vi "Main Loop.vi"(8 "error in (no error)":errorcluster, 10 "Chart Notifier":refnum<notifier>, 11 "Message Queues":T1) -> (0 "error out":errorcluster)   [LabVIEW 2018, in "Feed Module.lvlib" / "Feed Module Engine.lvlib"]
uses:
  Feed Module Engine.lvlib
  Feed Module/Controls/Feed Message Queues.ctl
  support/Message Queue/Message Cluster.ctl
  State Cluster.ctl
  State Enum.ctl
  Feed Module/Controls/Feed Module Settings Cluster.ctl
  Ismatec ISM 831C/Controls/Ismatech Settings Cluster.ctl
  Masterflex 7550-30/Controls/Settings Cluster.ctl
  Mettler Toledo/Controls/Settings Cluster.ctl
  Bronkhorst M13 Flow Meter/Settings Cluster.ctl
  PID 2 Parameters Cluster.ctl
  PID Input Enum.ctl
  PID 2 Output Enum.ctl
  Tacmina QI/Tacmina QI DAQ Setting.ctl
  KNF Pump/Settings Cluster plus SIMDOS.ctl
  ASIA Pump/Pump Settings.ctl
  VICI M50 Party Mode/Settings Cluster.ctl
  FLOM Pump/Settings Cluster.ctl
  SSI PR Class/SSI PR Settings Cluster.ctl
  PID 1 Parameters Cluster.ctl
  Feed Module/Controls/Feed Module Display.ctl
  Config Module/Controls/OP Window Display.ctl
  <vilib>/Platform/TimedLoop/XDataNode/timing_clust.ctl
  <vilib>/Platform/TimedLoop/XDataNode/nitl_modes.ctl
  <vilib>/Platform/TimedLoop/XDataNode/wakeup.ctl
  Tag VIs/Tag FGV Operation Enum.ctl
  support/Message Queue/Enqueue Message (Single).vi
  <vilib>/Utility/error.llb/Error Cluster From Error Code.vi
  <vilib>/Platform/TimedLoop/XDataNode/XDataNode.xnode
  <vilib>/ErrorRing/Error Ring.xnode
  support/Message Queue/Message Queue.lvlib
  <vilib>/Platform/TimedLoop/XDataNode/XDNodeRunTimeDep.lvlib
  Feed Module/Feed Module.lvlib
  Ismatec ISM 831C/Ismatec ISM 831C.lvlib
  Masterflex 7550-30/Masterflex 7550-30.lvlib
  Bronkhorst M13 Flow Meter/Bronkhorst M13 Flow Meter.lvlib
  Mettler Toledo/Mettler Toledo.lvlib
  Tacmina QI/Tacmina QI.lvlib
  Shared Variables/Dynamic Shared Variables.lvlib
  KNF Pump/KNF SIMDOS.lvlib
  ASIA Pump.lvlib
  VICI M50 Party Mode/VICI M6 M50 Party Mode.lvlib
  FLOM Pump/FLOM Pump.lvlib
  SSI PR Class/SSI PR Pump.lvlib
  support/Support Library.lvlib
panel:
  out "Period (s)":dbl format="%_4g"
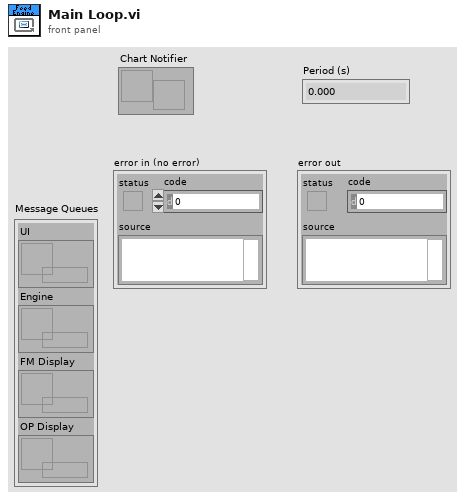
[diagram p1: front panel]
types:
  T1 = typedef "Feed Module.lvlib/Feed Message Queues.ctl" = cluster{"UI":refnum<queue>, "Engine":refnum<queue>, "FM Display":refnum<queue>, "OP Display":refnum<queue>}
  T2 = typedef "XDNodeRunTimeDep.lvlib/timing_clust.ctl" = cluster{"Expected End [f-1]":u64, "Actual End [f-1]":u64, "Finished Late? [f-1]":bool, "Expected End [i-1]":u64, "Actual End [i-1]":u64, "Finished Late? [i-1]":bool, "Expected Start [i]":u64, "Actual Start [i]":u64, "Expected Start [f]":u64, "Actual Start [f]":u64, "Source Name":string, "Structure Name":string, "Period":i64, "Deadline":i64, "Offset":i64, "Start":i64, "Priority":i32, "Timeout":i32, "Mode":T3, "Wakeup Reason":T4, "Error":errorcluster, "Source Type":string, "Secondary Source Type":string, "Global End Time":u64, "Global Start Time":u64, "Frame Duration":u64, "Iteration Duration":u64, "Assigned CPU":i32, "I/O Scan Engine Mode":u32}
  T3 = typedef "XDNodeRunTimeDep.lvlib/nitl_modes.ctl" = enum32{"No Change", "Process missed periods, maintain original phase", "Discard missed periods, maintain original phase", "Process missed periods, ignore original phase", "Discard missed periods, ignore original phase"}
  T4 = typedef "XDNodeRunTimeDep.lvlib/wakeup.ctl" = enum32{"Normal", "Aborted", "Asynchronous wakeup", "Timing source error", "Timed loop error", "Timeout"}
  T5 = cluster{"enable? (F)":bool, "name":string, "alarm on":bool, "priority":u32, "ack type":enum16{"Auto", "User", "None", "Each Occurrence"}, "area":string, "description":string, "log? (T)":bool}
  T6 = typedef "Tag FGV Operation Enum.ctl" = enum16{"Init", "Set Notification Queue", "Create Tag", "Commit", "Write Tag (Numeric)", "Write Tag (Boolean)", "Read All Tags", "Read One Tag", "Delete Tag Category", "Set Alarm Parameters (Numeric)", "Set Alarm Parameters (Boolean)", "Enable All Alarms", "Disable All Alarms", "Delete All Tags", "Read Alarms", "Ack Alarm"}
  T7 = enum32{"u32BitField", "bool", "double", "string", "int8", "uint8", "int16", "uint16", "int32", "uint32", "int64", "uint64", "single", "double waveform", "int16 waveform", "array of boolean", "array of int8", "array of uint8", "array of int16", "array of uint16", "array of int32", "array of uint32", "array of int64", "array of uint64", "array of single", "array of double", "array of double waveform", "array of int16 waveform", "array of string", "variant", "timestamp", "fixed point", "custom"}
  T8 = typedef "Feed Module.lvlib/Feed Module Engine.lvlib/State Enum.ctl" = enum16{"Measuring", "Idle", "Paused"}
  T9 = typedef "Feed Module.lvlib/OP Window Display.ctl" = cluster{"Flow":dbl, "Manual":dbl, "Pump Status":u16}
  T10 = typedef "Feed Module.lvlib/Feed Module Display.ctl" = cluster{"Flow":dbl, "Density":dbl, "FL Temp":dbl, "Scale Value":dbl, "Pump On?":enum16{"Off", "On", "Not Initialized"}, "Cycle Period":dbl, "Input Device":T11, "Output":T12, "Pump's Pressure":dbl, "Pump's Flow ":dbl}
  T11 = typedef "PID Input Enum.ctl" = enum16{"Default", "Bronkhorst M13", "Bronkhorst M14", "Scale Rate of Change"}
  T12 = typedef "PID 2 Output Enum.ctl" = enum16{"Default", "Ismatec ISM 831C", "Masterflex 7550-30", "VICI", "Tacmina QI", "KNF SIMDOS", "ASIA Type C", "FLOM UI-22-11", "SSI PR"}
  T13 = typedef "Feed Module.lvlib/Feed Module Engine.lvlib/State Cluster.ctl" = cluster{"State":T8, "Start Time":timestamp, "Configuration":T14, "Current Time":timestamp, "PID 1 Parameters":T26, "First Iteration":bool, "Data":cluster{"Flowmeter Output":dbl, "Density":dbl, "FL Temp":dbl, "Scale Output (g)":dbl, "Scale Rate of Change (g/min)":dbl, "PID 1 Output":dbl, "PID 2 Process Variable":dbl, "PID 2 output":dbl, "Pump Flow":dbl, "Pump Pressure":dbl}, "Process Name":string, "Pump On?":enum16{"Off", "On", "Not Initialized"}, "Input Error":bool, "Output Error":bool, "Log Started":bool, "Current Setpoint":dbl}
  T14 = typedef "Feed Module.lvlib/Feed Module Settings Cluster.ctl" = cluster{"Cycle Period":dbl, "Ismatech":T15, "Masterflex":T16, "Mettler":T17, "Bronkhorst M13 Flow Meter":T18, "PID 2 Parameters":T19, "Manual Entry":dbl, "Auto?":bool, "output range":cluster{"output high":dbl, "output low":dbl}, "Bronkhorst M14":T17, "Tacmina Settings":T20, "KNF SIMDOS Settings":T21, "ASIA Pump C":T22, "VICI Settings":T23, "FLOM Settings":T24, "SSI PR Settings":T25}
  T15 = typedef "Ismatec ISM 831C.lvlib/Ismatech Settings Cluster.ctl" = cluster{"VISA resource name":refnum<visa-resource-name>, "Simulated?":bool, "Pump Number":dbl, "Reverse?":bool}
  T16 = typedef "Masterflex 7550-30.lvlib/Settings Cluster.ctl" = cluster{"VISA resource name":refnum<visa-resource-name>, "Simulated?":bool, "Pump Number":dbl, "Reverse?":bool}
  T17 = typedef "Mettler Toledo.lvlib/Settings Cluster.ctl" = cluster{"VISA resource name":refnum<visa-resource-name>, "Simulated?":bool}
  T18 = typedef "Bronkhorst M13 Flow Meter.lvlib/Settings Cluster.ctl" = cluster{"VISA resource name":refnum<visa-resource-name>, "Simulated?":bool}
  T19 = typedef "PID 2 Parameters Cluster.ctl" = cluster{"Input Device":T11, "Output Device":T12, "Setpoint":dbl, "PID gains":cluster{"proportional gain (Kc)":dbl, "integral time (Ti, min)":dbl, "derivative time (Td, min)":dbl}}
  T20 = typedef "Tacmina QI.lvlib/Tacmina QI DAQ Setting.ctl" = cluster{"Analog DAQ Task":refnum<k21>, "Digital DAQ Task":refnum<k21>}
  T21 = typedef "KNF SIMDOS.lvlib/Settings Cluster plus SIMDOS.ctl" = cluster{"VISA resource name":refnum<visa-resource-name>, "Simulated?":bool}
  T22 = typedef "ASIA Pump.lvlib/Pump Settings.ctl" = cluster{"ASIA Pump #":i32, "channel":i32, "Simulated":bool}
  T23 = typedef "VICI M6 M50 Party Mode.lvlib/Settings Cluster.ctl" = cluster{"VISA resource name":refnum<visa-resource-name>, "Simulated?":bool, "Pump Letter":string, "Reverse?":bool}
  T24 = typedef "FLOM Pump.lvlib/Settings Cluster.ctl" = cluster{"VISA resource name":refnum<visa-resource-name>, "Simulated?":bool, "Pump Number":dbl}
  T25 = typedef "SSI PR Pump.lvlib/SSI PR Settings Cluster.ctl" = cluster{"VISA resource name":refnum<visa-resource-name>, "Simulated?":bool}
  T26 = typedef "PID 1 Parameters Cluster.ctl" = cluster{"Setpoint":dbl, "PID gains":cluster{"proportional gain (Kc)":dbl, "integral time (Ti, min)":dbl, "derivative time (Td, min)":dbl}}
  T27 = cluster{"Flowmeter Output":dbl, "Density":dbl, "FL Temp":dbl, "Scale Output (g)":dbl, "Scale Rate of Change (g/min)":dbl, "PID 1 Output":dbl, "PID 2 Process Variable":dbl, "PID 2 output":dbl, "Pump Flow":dbl, "Pump Pressure":dbl}
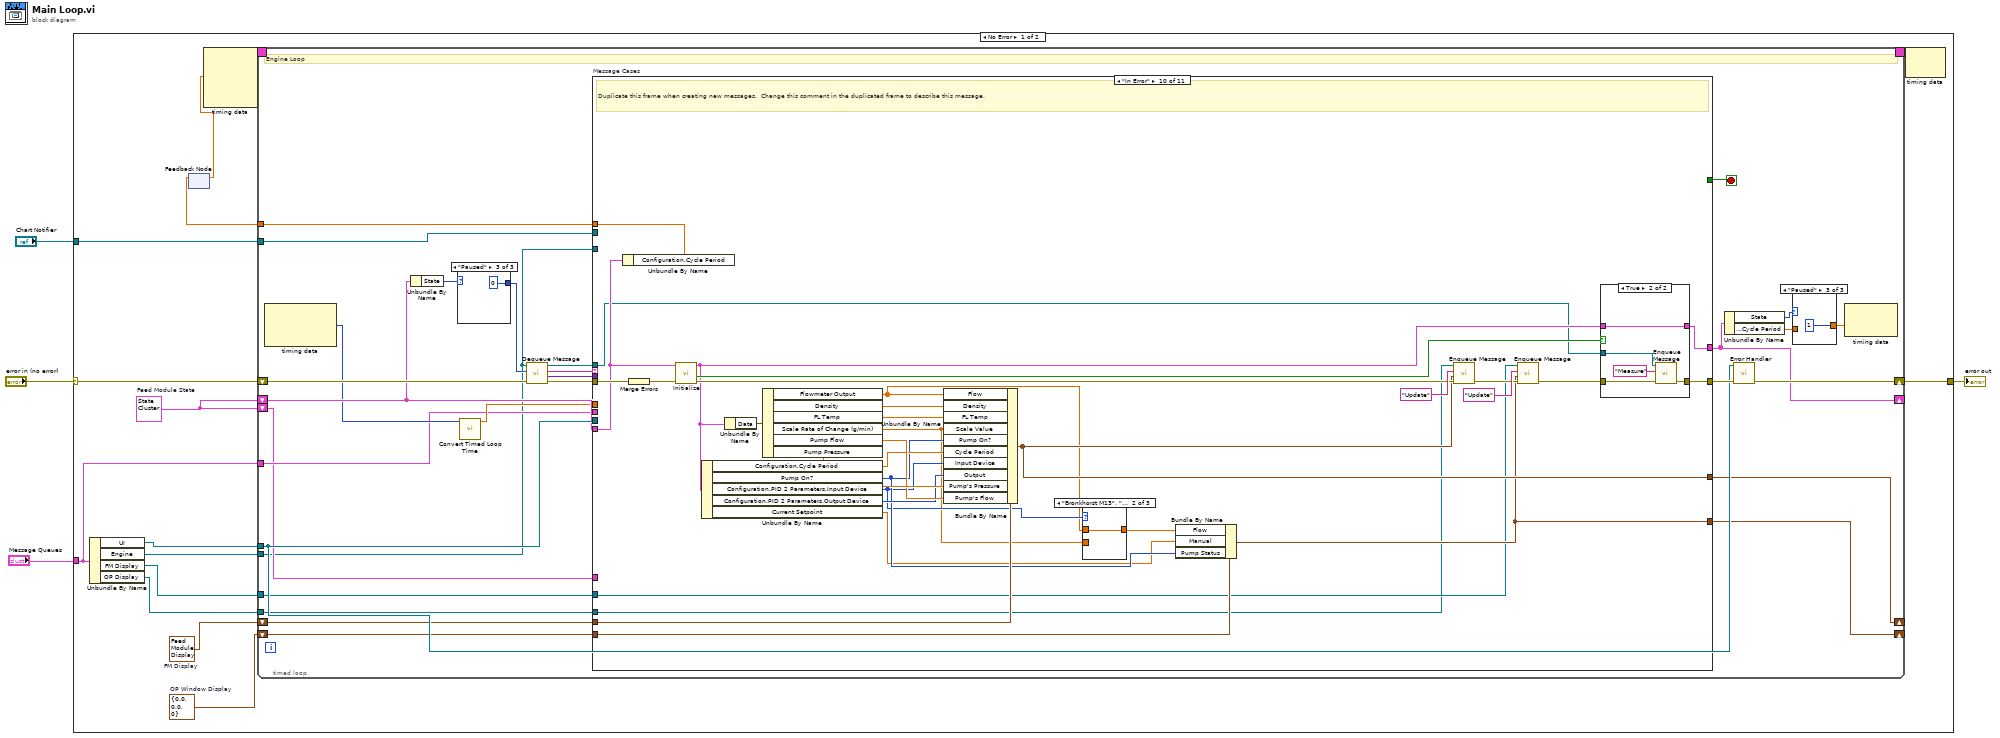
[diagram p0: block diagram]
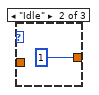
[diagram p3: hidden frame]
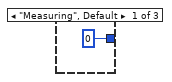
[diagram p4: hidden frame]
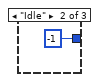
[diagram p5: hidden frame]
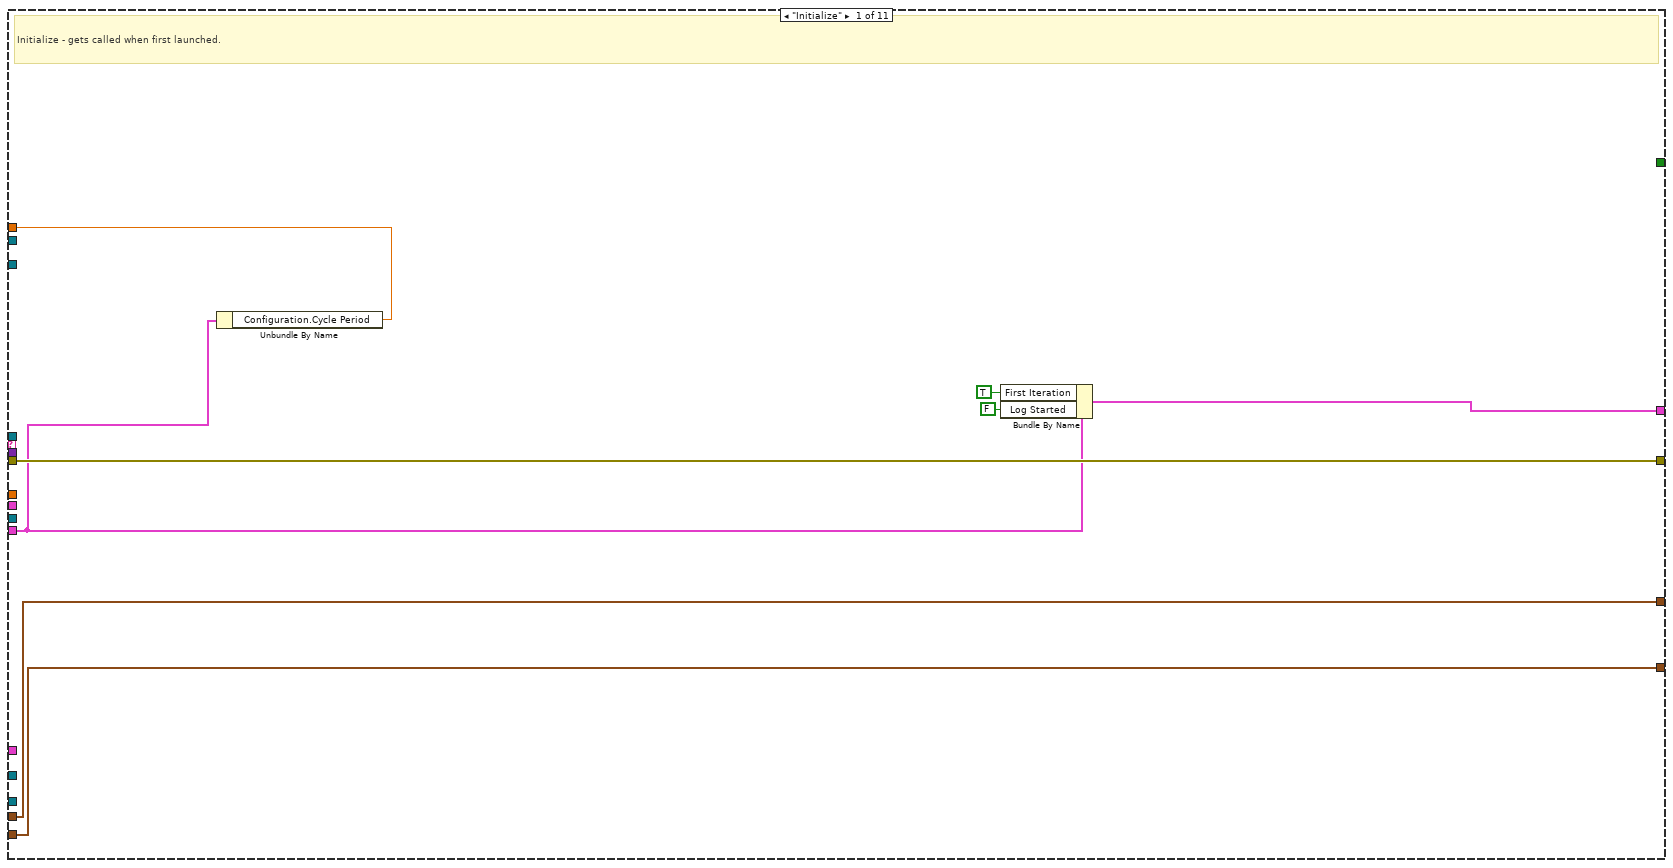
[diagram p6: hidden frame]
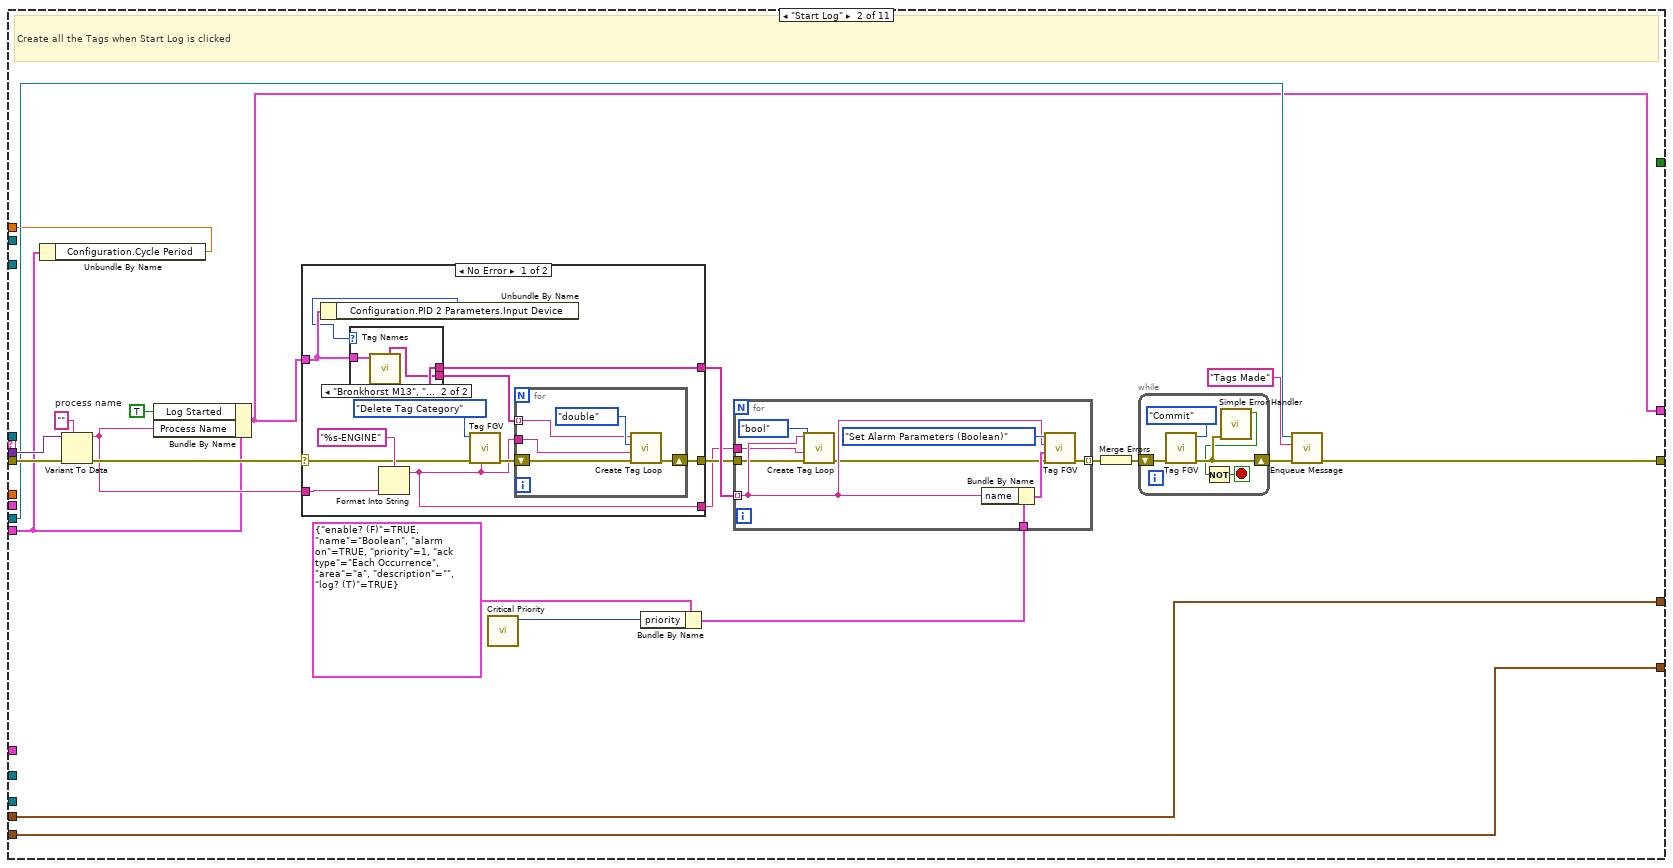
[diagram p7: hidden frame]
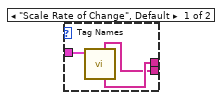
[diagram p8: hidden frame]
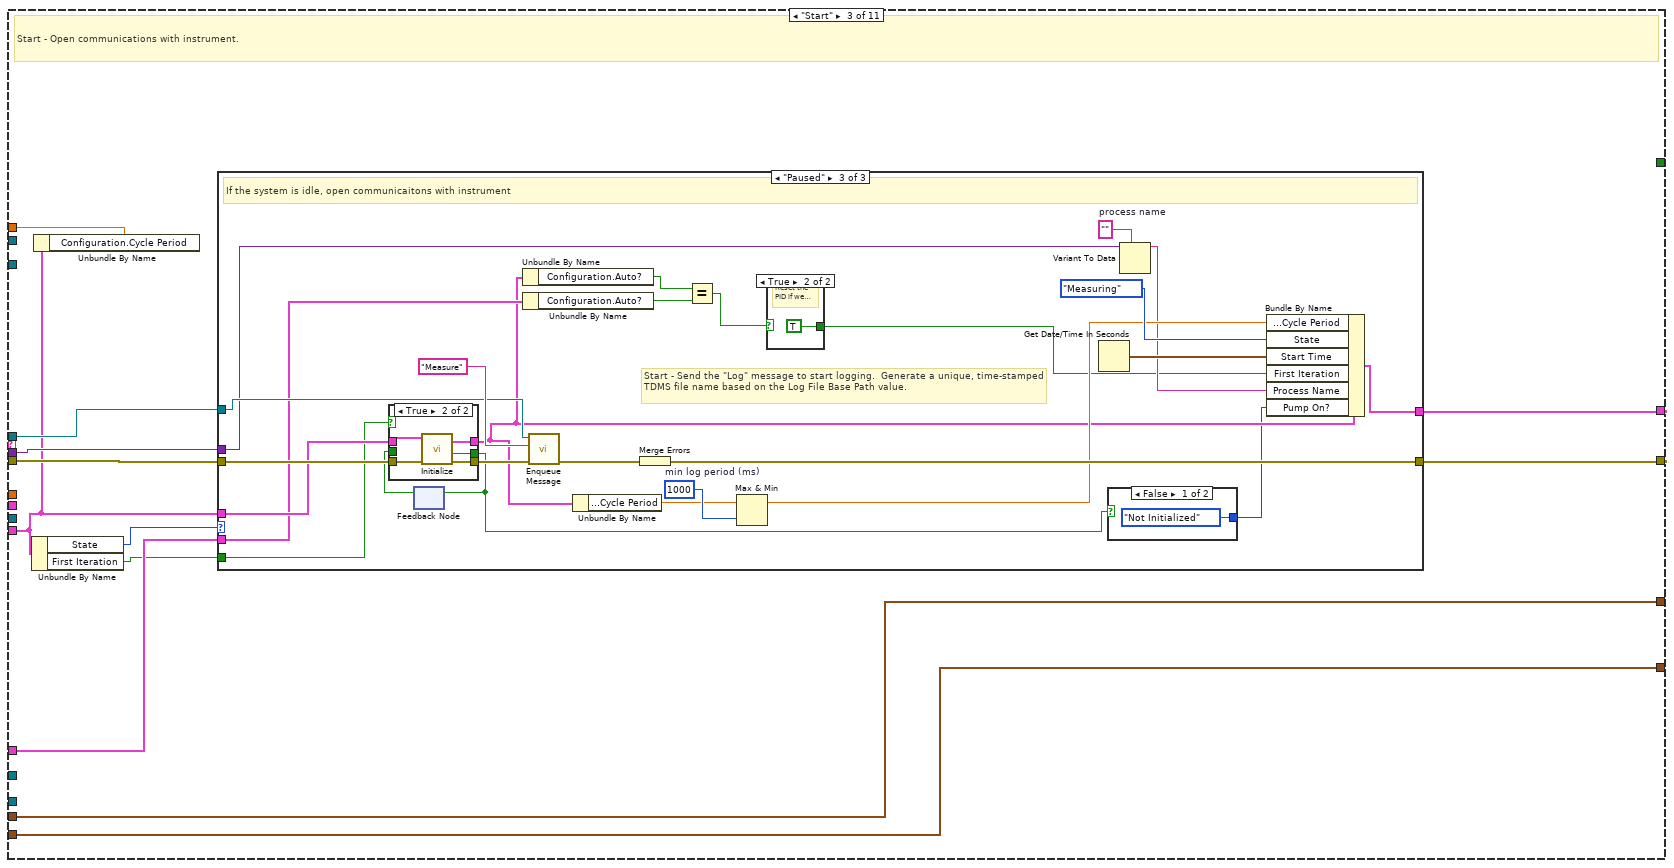
[diagram p10: hidden frame]
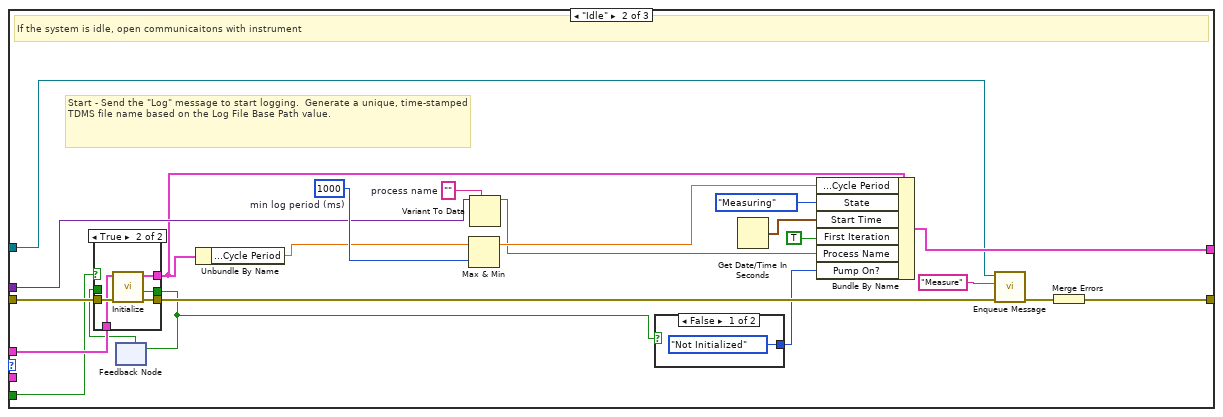
[diagram p12: hidden frame]
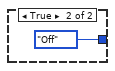
[diagram p14: hidden frame]
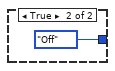
[diagram p16: hidden frame]
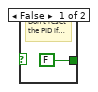
[diagram p17: hidden frame]
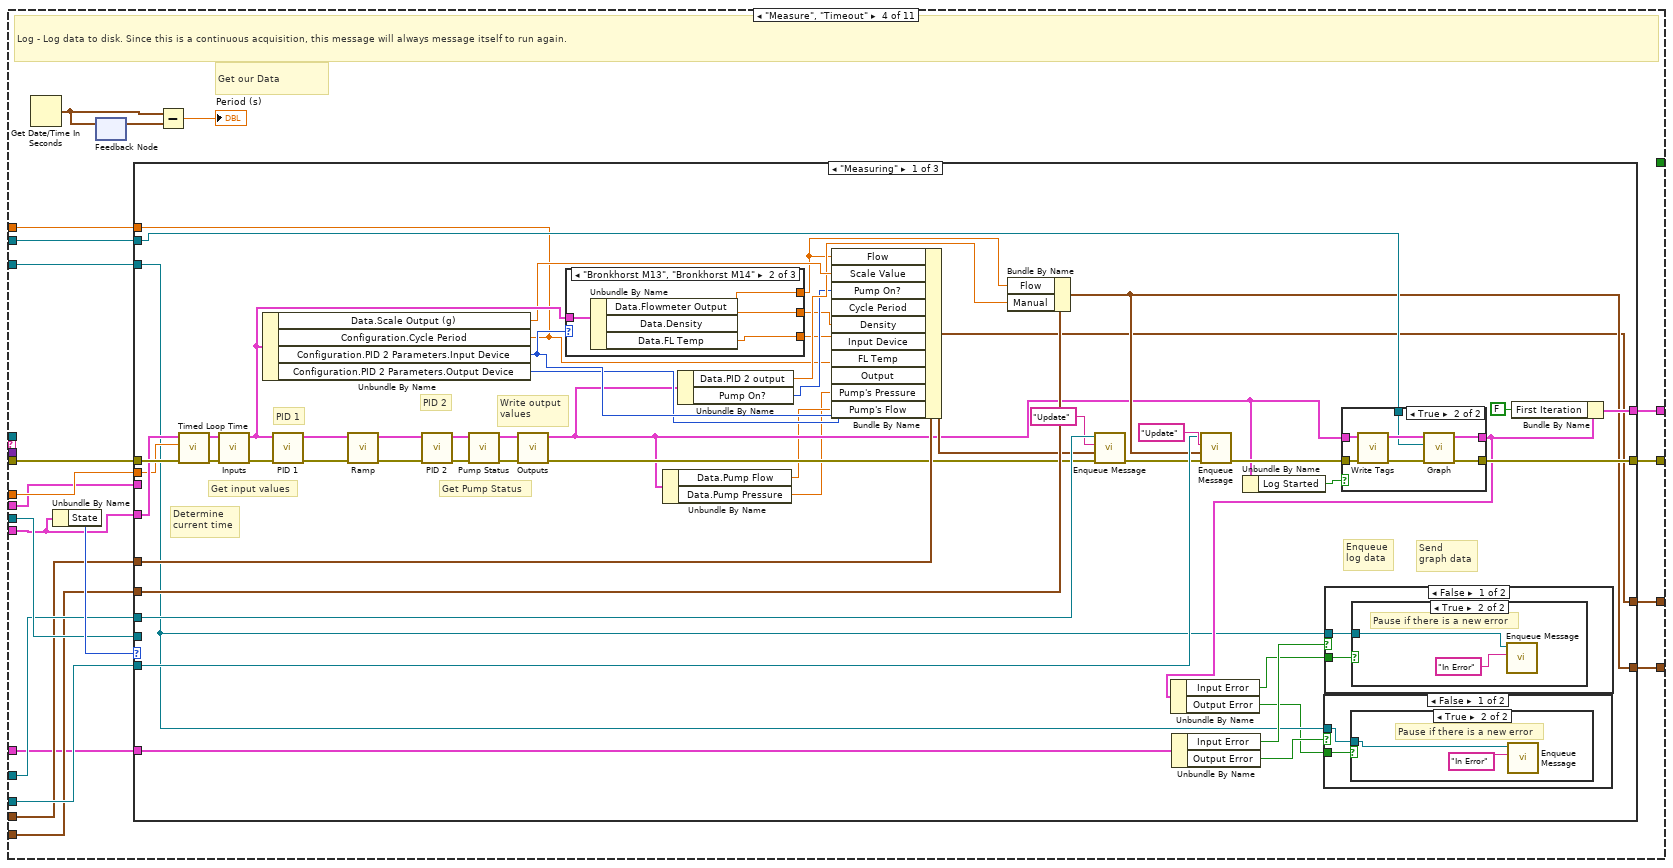
[diagram p18: hidden frame]
diagram:
  n1 = case shown="No Error" "error in (no error)" {
    selector: "error in (no error)" -> [w18 w566]
    tunnel: "Message Queues" -> [w14 _]
    tunnel: [w19 w566] -> w3
    tunnel: "Chart Notifier" -> [w12 _]
    frame No Error {
      w9 = T9 {"Flow"=0.0, "Manual"=0.0, "Pump Status"=0}  # OP Window Display
      w7 = T10 {"Flow"=0.0, "Density"=0.0, "FL Temp"=0.0, "Scale Value"=0.0, "Pump On?"=enum."Off", "Cycle Period"=500.0, "Input Device"=enum."Bronkhorst M13", "Output"=enum."Default", "Pump's Pressure"=0.0, "Pump's Flow "=0.0}  # FM Display
      w10 = T13 {"State"=enum."Idle", "Start Time"=timestamp(0 s since 1904-01-01), "Configuration"={"Cycle Period"=0.0, "Ismatech"={"VISA resource name"="", "Simulated?"=FALSE, "Pump Number"=1.0, "Reverse?"=FALSE}, "Masterflex"={"VISA resource name"="", "Simulated?"=FALSE, "Pump Number"=1.0, "Reverse?"=FALSE}, "Mettler"={"VISA resource name"="", "Simulated?"=FALSE}, "Bronkhorst M13 Flow Meter"={"VISA resource name"="", "Simulated?"=FALSE}, "PID 2 Parameters"={"Input Device"=enum."Bronkhorst M13", "Output Device"=enum."Ismatec ISM 831C", "Setpoint"=0.0, "PID gains"={"proportional gain (Kc)"=1.0, "integral time (Ti, min)"=0.01, "derivative time (Td, min)"=0.0}}, "Manual Entry"=0.0, "Auto?"=TRUE, "output range"={"output high"=100.0, "output low"=0.0}, "Bronkhorst M14"={"VISA resource name"="", "Simulated?"=FALSE}, "Tacmina Settings"={"Analog DAQ Task"="", "Digital DAQ Task"=""}, "KNF SIMDOS Settings"={"VISA resource name"="", "Simulated?"=TRUE}, "ASIA Pump C"={"ASIA Pump #"=0, "channel"=0, "Simulated"=FALSE}, "VICI Settings"={"VISA resource name"="", "Simulated?"=FALSE, "Pump Letter"="", "Reverse?"=FALSE}, "FLOM Settings"={"VISA resource name"="", "Simulated?"=TRUE, "Pump Number"=0.0}, "SSI PR Settings"={"VISA resource name"="", "Simulated?"=FALSE}}, "Current Time"=timestamp(0 s since 1904-01-01), "PID 1 Parameters"={"Setpoint"=0.0, "PID gains"={"proportional gain (Kc)"=1.0, "integral time (Ti, min)"=0.01, "derivative time (Td, min)"=0.0}}, "First Iteration"=FALSE, "Data"={"Flowmeter Output"=0.0, "Density"=0.0, "FL Temp"=0.0, "Scale Output (g)"=0.0, "Scale Rate of Change (g/min)"=0.0, "PID 1 Output"=0.0, "PID 2 Process Variable"=0.0, "PID 2 output"=0.0, "Pump Flow"=0.0, "Pump Pressure"=0.0}, "Process Name"="", "Pump On?"=enum."Off", "Input Error"=FALSE, "Output Error"=FALSE, "Log Started"=FALSE, "Current Setpoint"=0.0}  # Feed Module State
      n2 = Unbundle By Name(w14) -> ("UI"=w17:refnum<queue>, "Engine"=w13:refnum<queue>, "FM Display"=w11:refnum<queue>, "OP Display"=w8:refnum<queue>)
      n3 = feedback #1() -> (w5:dbl)  [unwired: 1 in]
      n4 = node-c288(w5) -> (w16:T2)  [unwired: 3 in]
      n5 = timed-loop {
        tunnel: w13 -> [w23]
        shift-right: [w37] -> _
        shift-left: w10 -> [w40]
        shift-right: [w42] -> w19
        shift-left: w18 -> [w48]
        tunnel: w17 -> [w41]
        timing: w16 -> [_]
        timing-out: [_] -> w15
        tunnel: w14 -> [w31]
        tunnel: w12 -> [w30]
        tunnel: w11 -> [w29]
        tunnel: w8 -> [w28]
        shift-right: [w27] -> _
        shift-left: w7 -> [w21]
        shift-right: [w26] -> _
        shift-left: w9 -> [w22]
        shift-left: w10 -> [w25]
        tunnel: [w20] -> w6
        stop <- w24 stop-if-true
        # "Engine Loop"
        n6 = node-c288() -> (w33:i64)  [unwired: 1 in, 2 out]
        n7 = Unbundle By Name(w40) -> ("State"=w39:T8)
        n8 = case shown="\"Paused\"" w39 {
          tunnel: [0 ("timeout in ms (-1)") -1 ("timeout in ms (-1)") 0 ("timeout in ms (-1)")] -> w38
          frame "Measuring", Default {
          }
          frame "Idle" {
          }
          frame "Paused" {
          }
        }
        n9 = call "Convert Timed Loop Time.vi"("Actual Start [i]"=w33) -> ("ET since start (s)"=w32:dbl)  [unwired: 10 in]
        n10 = call "Dequeue Message.vi"("error in (no error)"=w48, "timeout in ms (-1)"=w38, "Message Queue"=w23) -> ("error out"=w47:errorcluster, "Message Data"=w45:variant, "Message"=w46:string, "dup Message Queue"=w44:refnum<queue>)  [unwired: 5 in]
        n11 = case "Message Cases" shown="\"In Error\"" w46 {
          selector: w46 -> [_ _ _ _ _ _ _ _ _ _ w553]
          tunnel: w44 -> [_ _ w138 _ w413 _ _ w489 _ w502 _]
          tunnel: w47 -> [w67 w86 w137 w229 w400 w429 w481 w492 w501 w534 _]
          tunnel: [w67 w73 w139 w230 w405 w433 w475 w494 w500 w530 w554] -> w43
          tunnel: w40 -> [w61 w70 w129 w227 w399 w426 w477 w484 w497 w529 w550]
          tunnel: [w64 w72 w136 w228 w401 w431 w474 w484 w497 w531 w550] -> w37
          tunnel: [_ _ _ _ _ _ _ TRUE _ _ _] -> w24
          tunnel: w45 -> [_ w87 w134 _ _ _ w482 _ _ _ _]
          tunnel: w41 -> [_ w74 _ w231 w412 w442 _ w493 _ _ _]
          tunnel: w32 -> [_ _ _ w226 _ _ _ _ _ _ _]
          tunnel: w31 -> [_ _ _ w225 _ _ _ _ _ _ _]
          tunnel: w30 -> [_ _ _ w221 _ _ _ _ _ _ _]
          tunnel: w29 -> [_ _ _ w220 w403 w436 _ _ _ w504 _]
          tunnel: w28 -> [_ _ _ w219 w404 w435 _ _ _ w503 _]
          tunnel: w21 -> [w65 w90 w133 w218 w410 w440 w479 w486 w499 w522 w552]
          tunnel: [w65 w90 w133 w217 w410 w440 w479 w486 w499 w512 w552] -> w27
          tunnel: w22 -> [w66 w89 w132 w216 w402 w432 w478 w485 w498 w521 w551]
          tunnel: [w66 w89 w132 w215 w402 w432 w478 w485 w498 w505 w551] -> w26
          tunnel: w25 -> [_ _ w131 w214 _ _ _ _ _ _ _]
          tunnel: w23 -> [_ _ _ w213 _ _ _ _ _ _ _]
          tunnel: [w62 w71 w128 w212 w398 w425 w473 w483 w496 w528 w549] -> w20
          frame "Initialize" {
            # "Initialize - gets called when first launched."
            n12 = Unbundle By Name(w61) -> ("Configuration.Cycle Period"=w62:dbl)
            n13 = Bundle By Name(cluster=w61, "First Iteration"=TRUE, "Log Started"=FALSE) -> (w64:T13)
          }
          frame "Start Log" {
            w88 = ""  # process name
            # "Create all the Tags when Start Log is clicked"
            n14 = Unbundle By Name(w70) -> ("Configuration.Cycle Period"=w71:dbl)
            n15 = Variant To Data(error in=w86, type=w88, Variant=w87) -> (data=w84:string, error out=w85:errorcluster)
            n16 = Bundle By Name(cluster=w70, "Log Started"=TRUE, "Process Name"=w84) -> (w72:T13)
            n17 = case shown="No Error" w85 {
              selector: w85 -> [w112 w127]
              tunnel: [w115 w127] -> w79
              tunnel: w84 -> [w110 _]
              tunnel: [w109 _] -> w80
              tunnel: [w108 _] -> w77
              tunnel: w72 -> [w106 _]
              frame No Error {
                n18 = Unbundle By Name(w106) -> ("Configuration.PID 2 Parameters.Input Device"=w105:T11)
                n19 = case shown="\"Bronkhorst M13\", \"Bronkhorst M14\"" w105 {
                  tunnel: [w117 w121] -> w109
                  tunnel: [w116 w119] -> w107
                  tunnel: w106 -> [w118 w120]
                  frame "Scale Rate of Change", Default {
                    n20 = call "Tag Names.vi"("State in"=w118) -> ("All Boolean Tags"=w117:string[], "All  Numeric Tags"=w116:string[])  [unwired: 6 in, 3 out]
                  }
                  frame "Bronkhorst M13", "Bronkhorst M14" {
                    n21 = call "Tag Names.vi"("State in"=w120) -> ("All Boolean Tags"=w121:string[], "All  Numeric Tags"=w119:string[])  [unwired: 6 in, 3 out]
                  }
                }
                n22 = Format Into String(format string="%s-ENGINE", w110) -> (resulting string=w108:string)  [unwired: 2 in, 1 out]
                n23 = call "Tag FGV.vi"("Tag Category"=w108, "error in (no error)"=w112, "Operation"=Tag_FGV_Operation_Enum."Delete Tag Category") -> ("error out"=w111:errorcluster)  [unwired: 3 in, 5 out]
                n24 = for {
                  tunnel: w107 -> [w123] mode=indexing
                  shift-right: [w122] -> w115
                  shift-left: w111 -> [w125]
                  tunnel: w108 -> [w124]
                  n25 = call "Create Tag Loop.vi"("error in (no error)"=w125, "Tag Category"=w124, "data type"=T7."double", "Tag Name"=w123) -> ("error out"=w122:errorcluster)  [unwired: 7 in]
                }
              }
              frame Error {
              }
            }
            n26 = call "Critical Priority.vi"() -> ("critical priority"=w82:i32)  [unwired: 11 in]
            n27 = Bundle By Name(cluster=T5 {"enable? (F)"=TRUE, "name"="Boolean", "alarm on"=TRUE, "priority"=1, "ack type"=enum."Each Occurrence", "area"="a", "description"="", "log? (T)"=TRUE} ("Boolean alarm settings"), "priority"=w82) -> (w81:T5)
            n28 = for {
              tunnel: w81 -> [w104]
              tunnel: [w103] -> w78 mode=indexing
              tunnel: w80 -> [w99] mode=indexing
              tunnel: w79 -> [w97]
              tunnel: w77 -> [w98]
              n29 = call "Create Tag Loop.vi"("error in (no error)"=w97, "Tag Category"=w98, "data type"=T7."bool", "Tag Name"=w99) -> ("error out"=w96:errorcluster)  [unwired: 7 in]
              n30 = Bundle By Name(cluster=w104, "name"=w99) -> (w102:T5)
              n31 = call "Tag FGV.vi"("error in (no error)"=w96, "Data"=w102, "Tag Name"=w99, "Operation"=Tag_FGV_Operation_Enum."Set Alarm Parameters (Boolean)") -> ("error out"=w103:errorcluster)  [unwired: 2 in, 5 out]
            }
            n32 = Merge Errors(w78) -> (w69:errorcluster)
            n33 = while {
              shift-right: [w93] -> w68
              shift-left: w69 -> [w94]
              stop <- w91 stop-if-true
              n34 = call "Tag FGV.vi"("error in (no error)"=w94, "Operation"=Tag_FGV_Operation_Enum."Commit") -> ("error out"=w93:errorcluster)  [unwired: 4 in, 5 out]
              n35 = call <vilib>:"Simple Error Handler.vi"("error in (no error)"=w93) -> ("error?"=w92:bool)  [unwired: 4 in, 4 out]
              n36 = Not(x=w92) -> (.not. x?=w91:bool)
            }
            n37 = call-poly "Enqueue Message.vi"("error in (no error)"=w68, "Message"="Tags Made", "Message Queue"=w74) -> ("error out"=w73:errorcluster)  [unwired: 7 in, 1 out]
          }
          frame "Start" {
            # "Start - Open communications with instrument."
            n38 = Unbundle By Name(w129) -> ("State"=w135:T8, "First Iteration"=w130:bool)
            n39 = Unbundle By Name(w129) -> ("Configuration.Cycle Period"=w128:dbl)
            n40 = case shown="\"Paused\"" w135 {
              tunnel: [w140 w163 w199] -> w139
              tunnel: w138 -> [_ w154 w190]
              tunnel: w137 -> [w140 w152 w188]
              tunnel: w129 -> [w141 w151 w187]
              tunnel: [w141 w161 w197] -> w136
              tunnel: w134 -> [_ w149 w185]
              tunnel: w131 -> [_ _ w181]
              tunnel: w130 -> [_ w142 w176]
              frame "Measuring", Default {
                # "The system is already running. Ignore the \"Start\" message."
              }
              frame "Idle" {
                w150 = ""  # process name
                w158 = 1000  # min log period (ms)
                # "Start - Send the \"Log\" message to start logging.  Generate a unique, time-stamped TDMS file name based on the Log File Base Path value."
                # "If the system is idle, open communicaitons with instrument"
                n41 = feedback #2() -> (w144:bool)  [unwired: 1 in]
                n42 = case shown="True" w142 {
                  tunnel: w152 -> [w165 w171]
                  tunnel: w151 -> [w166 w170]
                  tunnel: [w166 w169] -> w147
                  tunnel: [w165 w168] -> w146
                  tunnel: [w164 w167] -> w143
                  tunnel: w144 -> [w164 _]
                  frame False {
                  }
                  frame True {
                    n43 = call "Initialize.vi"("error in (no error)"=w171, "State in"=w170) -> ("error out"=w168:errorcluster, "Pump Initialized"=w167:bool, "State out"=w169:T13)  [unwired: 7 in]
                  }
                }
                n44 = feedback-in #2(w143) -> ()
                n45 = Unbundle By Name(w147) -> ("Configuration.Cycle Period"=w157:dbl)
                n46 = Max & Min(x=w157, y=w158) -> (max(x,y)=w156:dbl)  [unwired: 1 out]
                n47 = Variant To Data(type=w150, Variant=w149) -> (data=w148:string)  [unwired: 1 in, 1 out]
                n48 = case shown="False" w143 {
                  tunnel: [enum16{"Off", "On", "Not Initialized"}."Not Initialized" ("Pump On?") enum16{"Off", "On", "Not Initialized"}."Off" ("Pump On?")] -> w145
                  frame False {
                  }
                  frame True {
                  }
                }
                n49 = Get Date/Time In Seconds() -> (seconds since 1Jan1904=w155:timestamp)
                n50 = Bundle By Name(cluster=w147, "Configuration.Cycle Period"=w156, "State"=State_Enum."Measuring", "Start Time"=w155, "First Iteration"=TRUE, "Process Name"=w148, "Pump On?"=w145) -> (w161:T13)
                n51 = call-poly "Enqueue Message.vi"("error in (no error)"=w146, "Message"="Measure", "Message Queue"=w154) -> ("error out"=w159:errorcluster)  [unwired: 7 in, 1 out]
                n52 = Merge Errors(w159) -> (w163:errorcluster)
              }
              frame "Paused" {
                w186 = ""  # process name
                w194 = 1000  # min log period (ms)
                # "Start - Send the \"Log\" message to start logging.  Generate a unique, time-stamped TDMS file name based on the Log File Base Path value."
                # "If the system is idle, open communicaitons with instrument"
                n53 = feedback #3() -> (w175:bool)  [unwired: 1 in]
                n54 = case shown="True" w176 {
                  tunnel: [w202 w207] -> w189
                  tunnel: w188 -> [w202 w206]
                  tunnel: w187 -> [w201 w205]
                  tunnel: [w201 w204] -> w178
                  tunnel: [w200 w203] -> w174
                  tunnel: w175 -> [w200 _]
                  frame False {
                  }
                  frame True {
                    n55 = call "Initialize.vi"("error in (no error)"=w206, "State in"=w205) -> ("error out"=w207:errorcluster, "Pump Initialized"=w203:bool, "State out"=w204:T13)  [unwired: 7 in]
                  }
                }
                n56 = feedback-in #3(w174) -> ()
                n57 = Unbundle By Name(w178) -> ("Configuration.Auto?"=w182:bool)
                n58 = Unbundle By Name(w181) -> ("Configuration.Auto?"=w180:bool)
                n59 = call-poly "Enqueue Message.vi"("error in (no error)"=w189, "Message"="Measure", "Message Queue"=w190) -> ("error out"=w195:errorcluster)  [unwired: 7 in, 1 out]
                n60 = Unbundle By Name(w178) -> ("Configuration.Cycle Period"=w193:dbl)
                n61 = Merge Errors(w195) -> (w199:errorcluster)
                n62 = Equal?(x=w182, y=w180) -> (x = y?=w183:bool)
                n63 = Max & Min(x=w193, y=w194) -> (max(x,y)=w192:dbl)  [unwired: 1 out]
                n64 = case shown="True" w183 {
                  tunnel: [FALSE ("First Iteration") TRUE ("First Iteration")] -> w179
                  frame False {
                    # "Don't reset the PID if we are switching Auto?"
                  }
                  frame True {
                    # "Reset the PID if we start from paused"
                  }
                }
                n65 = Get Date/Time In Seconds() -> (seconds since 1Jan1904=w191:timestamp)
                n66 = case shown="False" w174 {
                  tunnel: [enum16{"Off", "On", "Not Initialized"}."Not Initialized" ("Pump On?") enum16{"Off", "On", "Not Initialized"}."Off" ("Pump On?")] -> w177
                  frame False {
                  }
                  frame True {
                  }
                }
                n67 = Variant To Data(type=w186, Variant=w185) -> (data=w184:string)  [unwired: 1 in, 1 out]
                n68 = Bundle By Name(cluster=w178, "Configuration.Cycle Period"=w192, "State"=State_Enum."Measuring", "Start Time"=w191, "First Iteration"=w179, "Process Name"=w184, "Pump On?"=w177) -> (w197:T13)
              }
            }
          }
          frame "Measure", "Timeout" {
            # "Get our Data"
            # "Log - Log data to disk. Since this is a continuous acquisition, this message will always message itself to run again."
            n69 = Get Date/Time In Seconds() -> (seconds since 1Jan1904=w223:timestamp)
            n70 = Unbundle By Name(w227) -> ("State"=w232:T8)
            n71 = feedback-in #4(w223) -> ()
            n72 = feedback #4() -> (w224:timestamp)  [unwired: 1 in]
            n73 = case shown="\"Measuring\"" w232 {
              tunnel: w229 -> [w280 w315 w338]
              tunnel: w227 -> [w278 w313 w339]
              tunnel: w231 -> [_ _ _]
              tunnel: [w282 w314 w354] -> w230
              tunnel: [w275 w313 w333] -> w228
              tunnel: w226 -> [w276 _ w364]
              tunnel: w225 -> [_ _ _]
              tunnel: w221 -> [w273 _ w365]
              tunnel: w220 -> [w267 w318 w349]
              tunnel: w219 -> [w264 w319 w359]
              tunnel: w218 -> [w263 w317 w360]
              tunnel: [w253 w317 w358] -> w217
              tunnel: w216 -> [w262 w311 w361]
              tunnel: [w254 w311 w353] -> w215
              tunnel: w214 -> [w238 _ w348]
              tunnel: w213 -> [w249 _ w345]
              tunnel: [w237 w312 w324] -> w212
              frame "Measuring" {
                # "Get Pump Status"
                # "Send\ngraph data"
                # "Enqueue\nlog data"
                # "PID 2"
                # "PID 1"
                # "Determine\ncurrent time"
                # "Write output\nvalues"
                # "Get input values"
                n74 = call "Timed Loop Time.vi"("error in (no error)"=w280, "ET since start (s)"=w276, "State in"=w278) -> ("error out"=w281:errorcluster, "State out"=w279:T13)  [unwired: 7 in]
                n75 = call "Inputs.vi"("error in (no error)"=w281, "State in"=w279) -> ("error out"=w277:errorcluster, "State out"=w272:T13)  [unwired: 8 in]
                n76 = Unbundle By Name(w272) -> ("Data.Scale Output (g)"=w261:dbl, "Configuration.Cycle Period"=w237:dbl, "Configuration.PID 2 Parameters.Input Device"=w246:T11, "Configuration.PID 2 Parameters.Output Device"=w236:T12)
                n77 = call "PID 1.vi"("error in (no error)"=w277, "State in"=w272) -> ("error out"=w241:errorcluster, "State out"=w242:T13)  [unwired: 8 in]
                n78 = call "Ramp.vi"("error in (no error)"=w241, "State in"=w242) -> ("error out"=w240:errorcluster, "State Out"=w239:T13)  [unwired: 8 in]
                n79 = call "PID 2.vi"("error in (no error)"=w240, "State in"=w239) -> ("error out"=w269:errorcluster, "State out"=w271:T13)  [unwired: 8 in]
                n80 = call "Pump Status.vi"("error in (no error)"=w269, "State in"=w271) -> ("error out"=w268:errorcluster, "State out"=w270:T13)  [unwired: 8 in]
                n81 = call "Outputs.vi"("error in (no error)"=w268, "State in"=w270) -> ("error out"=w257:errorcluster, "State out"=w235:T13)  [unwired: 8 in]
                n82 = case shown="\"Bronkhorst M13\", \"Bronkhorst M14\"" w246 {
                  tunnel: w272 -> [_ w306 w310]
                  tunnel: [0.0 ("Scale Rate of Change (g/min)") w305 w309] -> w258
                  tunnel: [0.0 ("Density") w304 nan ("Density")] -> w245
                  tunnel: [0.0 ("Density") w303 nan ("Density")] -> w244
                  frame "Default", Default {
                  }
                  frame "Bronkhorst M13", "Bronkhorst M14" {
                    n83 = Unbundle By Name(w306) -> ("Data.Flowmeter Output"=w305:dbl, "Data.Density"=w304:dbl, "Data.FL Temp"=w303:dbl)
                  }
                  frame "Scale Rate of Change" {
                    n84 = Unbundle By Name(w310) -> ("Data.Scale Rate of Change (g/min)"=w309:dbl)
                  }
                }
                n85 = Unbundle By Name(w235) -> ("Data.Pump Flow"=w234:dbl, "Data.Pump Pressure"=w233:dbl)
                n86 = Unbundle By Name(w235) -> ("Data.PID 2 output"=w260:dbl, "Pump On?"=w259:enum16{"Off", "On", "Not Initialized"})
                n87 = Bundle By Name(cluster=w263, "Flow"=w258, "Scale Value"=w261, "Pump On?"=w259, "Cycle Period"=w237, "Density"=w245, "Input Device"=w246, "FL Temp"=w244, "Output"=w236, "Pump's Pressure"=w233, "Pump's Flow"=w234) -> (w253:T10)
                n88 = Bundle By Name(cluster=w262, "Flow"=w258, "Manual"=w260) -> (w254:T9)
                n89 = call-poly "Enqueue Message.vi"("error in (no error)"=w257, "Message Data"=w253, "Message"="Update", "Message Queue"=w267) -> ("error out"=w256:errorcluster)  [unwired: 6 in, 1 out]
                n90 = Unbundle By Name(w238) -> ("Input Error"=w252:bool, "Output Error"=w248:bool)
                n91 = call-poly "Enqueue Message.vi"("error in (no error)"=w256, "Message Data"=w254, "Message"="Update", "Message Queue"=w264) -> ("error out"=w255:errorcluster)  [unwired: 6 in, 1 out]
                n92 = Unbundle By Name(w235) -> ("Log Started"=w243:bool)
                n93 = case shown="True" w243 {
                  tunnel: [w284 w289] -> w282
                  tunnel: w273 -> [_ w288]
                  tunnel: w235 -> [w283 w287]
                  tunnel: w255 -> [w284 w286]
                  tunnel: [w283 w285] -> w250
                  frame False {
                  }
                  frame True {
                    n94 = call "Write Tags.vi"("error in (no error)"=w286, "State in"=w287) -> ("error out"=w290:errorcluster, "State out"=w291:T13)  [unwired: 8 in]
                    n95 = call "Graph.vi"("error in (no error)"=w290, "notifier out"=w288, "State in"=w291) -> ("error out"=w289:errorcluster, "State out"=w285:T13)  [unwired: 7 in]
                  }
                }
                n96 = Unbundle By Name(w250) -> ("Input Error"=w251:bool, "Output Error"=w247:bool)
                n97 = case shown="False" w248 {
                  tunnel: w247 -> [w293 _]
                  tunnel: w249 -> [w292 _]
                  frame False {
                    n98 = case shown="True" w293 {
                      tunnel: w292 -> [_ w295]
                      frame False {
                      }
                      frame True {
                        # "Pause if there is a new error"
                        n99 = call-poly "Enqueue Message.vi"("Message"="In Error", "Message Queue"=w295) -> ()  [unwired: 8 in, 2 out]
                      }
                    }
                  }
                  frame True {
                  }
                }
                n100 = case shown="False" w252 {
                  tunnel: w251 -> [w297 _]
                  tunnel: w249 -> [w296 _]
                  frame False {
                    n101 = case shown="True" w297 {
                      tunnel: w296 -> [_ w299]
                      frame False {
                      }
                      frame True {
                        # "Pause if there is a new error"
                        n102 = call-poly "Enqueue Message.vi"("Message"="In Error", "Message Queue"=w299) -> ()  [unwired: 8 in, 2 out]
                      }
                    }
                  }
                  frame True {
                  }
                }
                n103 = Bundle By Name(cluster=w250, "First Iteration"=FALSE) -> (w275:T13)
              }
              frame "Idle", Default {
                n104 = Unbundle By Name(w313) -> ("Configuration.Cycle Period"=w312:dbl)
                n105 = call-poly "Enqueue Message.vi"("error in (no error)"=w315, "Message Data"=w317, "Message"="Update", "Message Queue"=w318) -> ("error out"=w316:errorcluster)  [unwired: 6 in, 1 out]
                n106 = call-poly "Enqueue Message.vi"("error in (no error)"=w316, "Message Data"=w311, "Message"="Update", "Message Queue"=w319) -> ("error out"=w314:errorcluster)  [unwired: 6 in, 1 out]
              }
              frame "Paused" {
                # "PID is 0 when paused"
                # "Send\ngraph data"
                # "Enqueue\nlog data"
                n107 = call "Timed Loop Time.vi"("error in (no error)"=w338, "ET since start (s)"=w364, "State in"=w339) -> ("error out"=w366:errorcluster, "State out"=w367:T13)  [unwired: 7 in]
                n108 = call "Inputs.vi"("error in (no error)"=w366, "State in"=w367) -> ("error out"=w342:errorcluster, "State out"=w341:T13)  [unwired: 8 in]
                n109 = Bundle By Name(cluster=w341, "Data.PID 2 output"=0.0) -> (w331:T13)
                n110 = call "Outputs.vi"("error in (no error)"=w342, "State in"=w331) -> ("error out"=w336:errorcluster, "State out"=w337:T13)  [unwired: 8 in]
                n111 = call "Pump Status.vi"("error in (no error)"=w336, "State in"=w337) -> ("error out"=w335:errorcluster, "State out"=w327:T13)  [unwired: 8 in]
                n112 = Unbundle By Name(w327) -> ("Log Started"=w326:bool)
                n113 = case shown="True" w326 {
                  tunnel: w365 -> [_ w374]
                  tunnel: [w368 w373] -> w356
                  tunnel: w327 -> [w369 w372]
                  tunnel: w335 -> [w368 w371]
                  tunnel: [w369 w370] -> w334
                  frame False {
                  }
                  frame True {
                    n114 = call "Write Tags.vi"("error in (no error)"=w371, "State in"=w372) -> ("error out"=w376:errorcluster, "State out"=w375:T13)  [unwired: 8 in]
                    n115 = call "Graph.vi"("error in (no error)"=w376, "notifier out"=w374, "State in"=w375) -> ("error out"=w373:errorcluster, "State out"=w370:T13)  [unwired: 7 in]
                  }
                }
                n116 = Unbundle By Name(w327) -> ("Pump On?"=w351:enum16{"Off", "On", "Not Initialized"})
                n117 = Bundle By Name(cluster=w334, "First Iteration"=FALSE) -> (w333:T13)
                n118 = Unbundle By Name(w331) -> ("Data.Scale Output (g)"=w357:dbl, "Configuration.PID 2 Parameters.Input Device"=w325:T11, "Configuration.Cycle Period"=w324:dbl, "Data.PID 2 output"=w352:dbl, "Data.Pump Flow"=w323:dbl, "Data.Pump Pressure"=w322:dbl)
                n119 = case shown="\"Bronkhorst M13\", \"Bronkhorst M14\"" w325 {
                  tunnel: w331 -> [_ w383 w387]
                  tunnel: [0.0 ("Scale Rate of Change (g/min)") w382 w386] -> w330
                  tunnel: [0.0 ("Density") w381 nan ("Density")] -> w329
                  tunnel: [0.0 ("Density") w380 nan ("Density")] -> w328
                  frame "Default", Default {
                  }
                  frame "Bronkhorst M13", "Bronkhorst M14" {
                    n120 = Unbundle By Name(w383) -> ("Data.Flowmeter Output"=w382:dbl, "Data.Density"=w381:dbl, "Data.FL Temp"=w380:dbl)
                  }
                  frame "Scale Rate of Change" {
                    n121 = Unbundle By Name(w387) -> ("Data.Scale Rate of Change (g/min)"=w386:dbl)
                  }
                }
                n122 = Bundle By Name(cluster=w360, "Flow"=w330, "Scale Value"=w357, "Pump On?"=w351, "Cycle Period"=w324, "Density"=w329, "FL Temp"=w328, "Input Device"=w325, "Pump's Pressure"=w322, "Pump's Flow"=w323) -> (w358:T10)
                n123 = case shown="\"Off\", Default" w351 {
                  tunnel: w352 -> [_ w397]
                  tunnel: [0.0 w397] -> w350
                  frame "Off", Default {
                  }
                  frame "On" {
                  }
                }
                n124 = call-poly "Enqueue Message.vi"("error in (no error)"=w356, "Message Data"=w358, "Message"="Update", "Message Queue"=w349) -> ("error out"=w355:errorcluster)  [unwired: 6 in, 1 out]
                n125 = Unbundle By Name(w333) -> ("Input Error"=w346:bool, "Output Error"=w343:bool)
                n126 = Unbundle By Name(w348) -> ("Input Error"=w347:bool, "Output Error"=w344:bool)
                n127 = Bundle By Name(cluster=w361, "Flow"=w330, "Manual"=w350) -> (w353:T9)
                n128 = case shown="False" w344 {
                  tunnel: w343 -> [w389 _]
                  tunnel: w345 -> [w388 _]
                  frame False {
                    n129 = case shown="True" w389 {
                      tunnel: w388 -> [_ w391]
                      frame False {
                      }
                      frame True {
                        n130 = call-poly "Enqueue Message.vi"("Message"="In Error", "Message Queue"=w391) -> ()  [unwired: 8 in, 2 out]
                      }
                    }
                  }
                  frame True {
                  }
                }
                n131 = case shown="False" w347 {
                  tunnel: w346 -> [w393 _]
                  tunnel: w345 -> [w392 _]
                  frame False {
                    n132 = case shown="True" w393 {
                      tunnel: w392 -> [_ w395]
                      frame False {
                      }
                      frame True {
                        n133 = call-poly "Enqueue Message.vi"("Message"="In Error", "Message Queue"=w395) -> ()  [unwired: 8 in, 2 out]
                      }
                    }
                  }
                  frame True {
                  }
                }
                n134 = call-poly "Enqueue Message.vi"("error in (no error)"=w355, "Message Data"=w353, "Message"="Update", "Message Queue"=w359) -> ("error out"=w354:errorcluster)  [unwired: 6 in, 1 out]
              }
            }
            n135 = Subtract(x=w223, y=w224) -> (x-y=→"Period (s)":dbl)
          }
          frame "Stop" {
            # "Stop - Flush the message queue of any pending \"Log\" messages. Call 'Flush Data to Log File.vi' so any pending data is not lost."
            n136 = Unbundle By Name(w399) -> ("State"=w411:T8)
            n137 = Unbundle By Name(w399) -> ("Configuration.Cycle Period"=w398:dbl)
            n138 = case shown="\"Measuring\", Default" w411 {
              tunnel: [w418 w424] -> w406
              tunnel: w400 -> [w414 w424]
              tunnel: w413 -> [_ _]
              tunnel: w412 -> [w422 _]
              tunnel: w399 -> [w416 w423]
              tunnel: [w420 w423] -> w401
              frame "Measuring", Default {
                # "If the system is logging, stop logging."
                n139 = call "Close.vi"("error in (no error)"=w414, "State in"=w416) -> ("error out"=w415:errorcluster, "State out"=w417:T13)  [unwired: 8 in]
                n140 = Bundle By Name(cluster=w417, "State"=State_Enum."Idle") -> (w420:T13)
                n141 = call-poly "Enqueue Message.vi"("error in (no error)"=w415, "Message"="Logging Stopped", "Message Queue"=w422) -> ("error out"=w418:errorcluster)  [unwired: 7 in, 1 out]
              }
              frame "Idle" {
                # "The system is already idle. Ignore the \"Stop\" message."
              }
            }
            n142 = call-poly "Enqueue Message.vi"("error in (no error)"=w406, "Message Data"=w401, "Message"="Update", "Message Queue"=w403) -> ("error out"=w407:errorcluster)  [unwired: 6 in, 1 out]
            n143 = call-poly "Enqueue Message.vi"("error in (no error)"=w407, "Message Data"=w402, "Message"="Update", "Message Queue"=w404) -> ("error out"=w405:errorcluster)  [unwired: 6 in, 1 out]
          }
          frame "Pause" {
            # "Stop - Flush the message queue of any pending \"Log\" messages. Call 'Flush Data to Log File.vi' so any pending data is not lost."
            n144 = Unbundle By Name(w426) -> ("State"=w441:T8, "First Iteration"=w430:bool)
            n145 = Unbundle By Name(w426) -> ("Configuration.Cycle Period"=w425:dbl)
            n146 = case shown="True" w430 {
              tunnel: w426 -> [w444 w449]
              tunnel: [w444 w450] -> w427
              tunnel: w429 -> [w443 w447]
              tunnel: [w443 w446] -> w428
              frame False {
              }
              frame True {
                # "If we load to a paused state we initialize"
                n147 = call "Initialize.vi"("error in (no error)"=w447, "State in"=w449) -> ("error out"=w446:errorcluster, "Pump Initialized"=w451:bool, "State out"=w448:T13)  [unwired: 7 in]
                n148 = case shown="True" w451 {
                  tunnel: [enum16{"Off", "On", "Not Initialized"}."Not Initialized" ("Pump On?") enum16{"Off", "On", "Not Initialized"}."Off" ("Pump On?")] -> w452
                  tunnel: [_ FALSE] -> w445
                  frame False {
                  }
                  frame True {
                  }
                }
                n149 = Bundle By Name(cluster=w448, "Pump On?"=w452, "First Iteration"=w445) -> (w450:T13)
              }
            }
            n150 = case shown="\"Measuring\", Default" w441 {
              tunnel: [w460 w468 w472] -> w434
              tunnel: w428 -> [w458 w468 w472]
              tunnel: w442 -> [w464 _ _]
              tunnel: w427 -> [w459 w466 w470]
              tunnel: [w462 w465 w469] -> w431
              frame "Measuring", Default {
                # "If the system is logging, stop logging."
                n151 = call "Pause.vi"("error in (no error)"=w458, "State in"=w459) -> ("error out"=w457:errorcluster, "State out"=w456:T13)  [unwired: 8 in]
                n152 = Bundle By Name(cluster=w456, "State"=State_Enum."Paused") -> (w462:T13)
                n153 = call-poly "Enqueue Message.vi"("error in (no error)"=w457, "Message"="Logging Stopped", "Message Queue"=w464) -> ("error out"=w460:errorcluster)  [unwired: 7 in, 1 out]
              }
              frame "Idle" {
                # "The system is already idle. Ignore the \"Stop\" message."
                n154 = Bundle By Name(cluster=w466, "State"=State_Enum."Paused") -> (w465:T13)
              }
              frame "Paused" {
                n155 = Bundle By Name(cluster=w470, "State"=State_Enum."Paused") -> (w469:T13)
              }
            }
            n156 = call-poly "Enqueue Message.vi"("error in (no error)"=w434, "Message Data"=w431, "Message"="Update", "Message Queue"=w436) -> ("error out"=w437:errorcluster)  [unwired: 6 in, 1 out]
            n157 = call-poly "Enqueue Message.vi"("error in (no error)"=w437, "Message Data"=w432, "Message"="Update", "Message Queue"=w435) -> ("error out"=w433:errorcluster)  [unwired: 6 in, 1 out]
          }
          frame "Update Settings" {
            w480 = T14 {"Cycle Period"=0.0, "Ismatech"={"VISA resource name"="", "Simulated?"=FALSE, "Pump Number"=1.0, "Reverse?"=FALSE}, "Masterflex"={"VISA resource name"="", "Simulated?"=FALSE, "Pump Number"=1.0, "Reverse?"=FALSE}, "Mettler"={"VISA resource name"="", "Simulated?"=FALSE}, "Bronkhorst M13 Flow Meter"={"VISA resource name"="", "Simulated?"=FALSE}, "PID 2 Parameters"={"Input Device"=enum."Bronkhorst M13", "Output Device"=enum."Ismatec ISM 831C", "Setpoint"=0.0, "PID gains"={"proportional gain (Kc)"=1.0, "integral time (Ti, min)"=0.01, "derivative time (Td, min)"=0.0}}, "Manual Entry"=0.0, "Auto?"=TRUE, "output range"={"output high"=100.0, "output low"=0.0}, "Bronkhorst M14"={"VISA resource name"="", "Simulated?"=FALSE}, "Tacmina Settings"={"Analog DAQ Task"="", "Digital DAQ Task"=""}, "KNF SIMDOS Settings"={"VISA resource name"="", "Simulated?"=TRUE}, "ASIA Pump C"={"ASIA Pump #"=0, "channel"=0, "Simulated"=FALSE}, "VICI Settings"={"VISA resource name"="", "Simulated?"=FALSE, "Pump Letter"="", "Reverse?"=FALSE}, "FLOM Settings"={"VISA resource name"="", "Simulated?"=TRUE, "Pump Number"=0.0}, "SSI PR Settings"={"VISA resource name"="", "Simulated?"=FALSE}}  # Configuration
            # "New settings are available, update the current ones stored in the shift register with the settings sent as part of the message"
            n158 = Variant To Data(error in=w481, type=w480, Variant=w482) -> (data=w476:T14, error out=w475:errorcluster)
            n159 = Bundle By Name(cluster=w477, "Configuration"=w476) -> (w474:T13)
            n160 = Unbundle By Name(w474) -> ("Configuration.Cycle Period"=w473:dbl)
          }
          frame "Exit" {
            # "Release the Logging queue reference"
            # "Don't check the error out. The UI message queue may have already been released."
            # "Stop the VI"
            # "Exit - Send the Exit message to the UI Message Handler.  Call 'Flush Data to Log File.vi' so any pending data is not lost."
            n161 = Release Queue(queue=w489, error in (no error)=w492) -> (error out=w488:errorcluster)  [unwired: 1 in, 2 out]
            n162 = call-poly "Enqueue Message.vi"("Priority Message? (F)"=TRUE, "Message"="Exit", "Message Queue"=w493) -> ("error out"=w487:errorcluster)  [unwired: 7 in, 1 out]
            n163 = call <vilib>:"Clear Errors.vi"("error in (no error)"=w487) -> ()  [unwired: 5 in, 2 out]
            n164 = Unbundle By Name(w484) -> ("Configuration.Cycle Period"=w483:dbl)
            n165 = Merge Errors(w488) -> (w494:errorcluster)
          }
          frame "---Copy This Frame---" {
            # "Duplicate this frame when creating new messages.  Change this comment in the duplicated frame to describe this message."
            n166 = Merge Errors(w501) -> (w500:errorcluster)
            n167 = Unbundle By Name(w497) -> ("Configuration.Cycle Period"=w496:dbl)
          }
          frame "In Error" {
            # "Duplicate this frame when creating new messages.  Change this comment in the duplicated frame to describe this message."
            n168 = Unbundle By Name(w529) -> ("Configuration.Cycle Period"=w528:dbl)
            n169 = Merge Errors(w534) -> (w532:errorcluster)
            n170 = call "Initialize.vi"("error in (no error)"=w532, "State in"=w529) -> ("error out"=w526:errorcluster, "Pump Initialized"=w533:bool, "State out"=w515:T13)  [unwired: 7 in]
            n171 = Unbundle By Name(w515) -> ("Configuration.Cycle Period"=w514:dbl, "Pump On?"=w511:enum16{"Off", "On", "Not Initialized"}, "Configuration.PID 2 Parameters.Input Device"=w509:T11, "Configuration.PID 2 Parameters.Output Device"=w513:T12, "Current Setpoint"=w510:dbl)
            n172 = Unbundle By Name(w515) -> ("Data"=w520:T27)
            n173 = Unbundle By Name(w520) -> ("Flowmeter Output"=w508:dbl, "Density"=w519:dbl, "FL Temp"=w518:dbl, "Scale Rate of Change (g/min)"=w507:dbl, "Pump Flow"=w516:dbl, "Pump Pressure"=w517:dbl)
            n174 = Bundle By Name(cluster=w522, "Flow"=w508, "Density"=w519, "FL Temp"=w518, "Scale Value"=w507, "Pump On?"=w511, "Cycle Period"=w514, "Input Device"=w509, "Output"=w513, "Pump's Pressure"=w517, "Pump's Flow"=w516) -> (w512:T10)
            n175 = case shown="\"Bronkhorst M13\", \"Bronkhorst M14\"" w509 {
              tunnel: w508 -> [_ w536 _]
              tunnel: w507 -> [_ _ w537]
              tunnel: [0.0 ("Scale Rate of Change (g/min)") w536 w537] -> w506
              frame "Default", Default {
              }
              frame "Bronkhorst M13", "Bronkhorst M14" {
              }
              frame "Scale Rate of Change" {
              }
            }
            n176 = Bundle By Name(cluster=w521, "Flow"=w506, "Manual"=w510, "Pump Status"=w511) -> (w505:T9)
            n177 = call-poly "Enqueue Message.vi"("error in (no error)"=w526, "Message Data"=w512, "Message"="Update", "Message Queue"=w503) -> ("error out"=w524:errorcluster)  [unwired: 6 in, 1 out]
            n178 = call-poly "Enqueue Message.vi"("error in (no error)"=w524, "Message Data"=w505, "Message"="Update", "Message Queue"=w504) -> ("error out"=w523:errorcluster)  [unwired: 6 in, 1 out]
            n179 = case shown="True" w533 {
              tunnel: w502 -> [w542 w546]
              tunnel: w523 -> [w541 w545]
              tunnel: [w539 w548] -> w531
              tunnel: w515 -> [w539 w548]
              tunnel: [w538 w544] -> w530
              frame False {
                n180 = Wait (ms)(milliseconds to wait=u32 5000) -> ()  [unwired: 1 out]
                n181 = call-poly "Enqueue Message.vi"("error in (no error)"=w541, "Message"="In Error", "Message Queue"=w542) -> ("error out"=w538:errorcluster)  [unwired: 7 in, 1 out]
              }
              frame True {
                n182 = call-poly "Enqueue Message.vi"("error in (no error)"=w545, "Message"="Measure", "Message Queue"=w546) -> ("error out"=w544:errorcluster)  [unwired: 7 in, 1 out]
              }
            }
          }
          frame Default {
            # "'Default' case only runs if there is a message that isn't defined in any of the other cases.  Output a programming error."
            n183 = Unbundle By Name(w550) -> ("Configuration.Cycle Period"=w549:dbl)
            n184 = xnode "Error Ring"("parameter 0"=w553) -> ("error out"=w554:errorcluster)
          }
        }
        n185 = Unbundle By Name(w37) -> ("State"=w36:T8, "Configuration.Cycle Period"=w34:dbl)
        n186 = call "Error Handler.vi"("error in (no error)"=w43, "Message Queue"=w41) -> ("dup error in"=w42:errorcluster)  [unwired: 8 in, 1 out]
        n187 = case shown="\"Paused\"" w36 {
          tunnel: [w49 1 1] -> w35
          tunnel: w34 -> [w49 _ _]
          frame "Measuring" {
          }
          frame "Idle" {
          }
          frame "Paused" {
          }
        }
        n188 = node-c288(w35) -> ()  [unwired: 1 in, 1 out]
      }
      n189 = feedback-in #1(w6) -> ()
      n190 = node-c288(w15) -> ()  [unwired: 1 out]
    }
    frame Error {
    }
  }
  "error out" <- w3
